vi "remove channel action.vi"(6 "user event":T1, 7 "channel":i32, 8 "error in":errorcluster, 9 "channel list":refnum<vi>, 10 "engine configuration in":refnum<class "engine configuration.lvclass">, 11 "io configuration in":refnum<class "io configuration.lvclass">) -> (0 "error out":errorcluster, 2 "engine configuration out":refnum<class "engine configuration.lvclass">, 3 "io configuration out":refnum<class "io configuration.lvclass">)   [LabVIEW 2014, in "io editor node.lvclass"]
uses:
  io editor node.lvclass
  <vilib>/NI/Configuration Framework/Controls/EventCluster.ctl
  <vilib>/NI/Configuration Framework/NISE_CEF_TreeControl.lvlib
  <vilib>/NI/Module Execution Interface/Engine Configuration/engine configuration.lvclass
  <vilib>/NI/Configuration Framework/serializable configuration/NISE_CEF_serializable configuration.lvclass
  configuration/io configuration.lvclass
  <vilib>/NI/Configuration Framework/Node/UserEventRef.ctl
  <vilib>/NI/Configuration Framework/Node/NISE_CEF_Node.lvclass
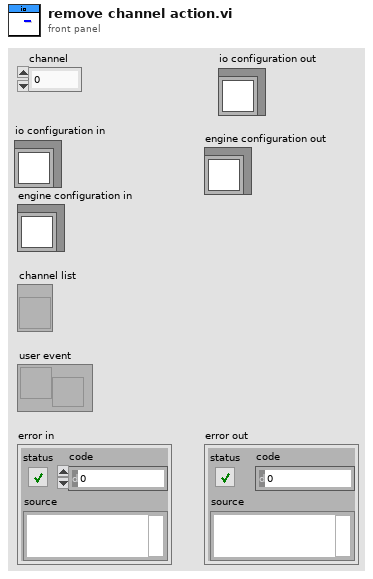
[diagram p1: front panel]
types:
  T1 = typedef "NISE_CEF_Node.lvclass/UserEventRef.ctl" = refnum<user-event>
  T2 = typedef "io editor node.lvclass/table line.ctl" = cluster{"channel":refnum<class "TBM channel.lvclass">, "tag name":string}
  T3 = typedef "NISE_CEF_TreeControl.lvlib/EventCluster.ctl" = cluster{"command":string, "data":string}
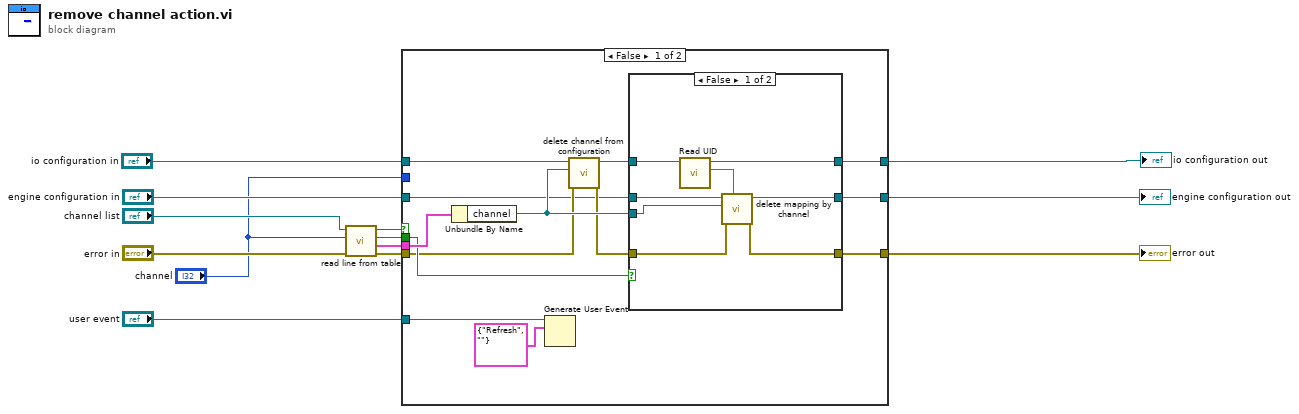
[diagram p0: block diagram]
diagram:
  n1 = call "read line from table.vi"("error in"="error in", "line number"="channel", "channels table"="channel list") -> ("error out"=w9:errorcluster, "line"=w5:T2, "empty tag?"=w8:bool, "empty channel?"=w7:bool)  [unwired: 5 in]
  n2 = case shown="False" w7 {
    tunnel: [w16 w39] -> w3
    tunnel: "channel" -> [_ _]
    tunnel: w5 -> [w26 _]
    tunnel: "io configuration in" -> [w24 w38]
    tunnel: "engine configuration in" -> [w19 w40]
    tunnel: w8 -> [w25 _]
    tunnel: w9 -> [w22 w39]
    tunnel: [w18 w40] -> w11
    tunnel: [w17 w38] -> w1
    tunnel: "user event" -> [w14 _]
    frame False {
      n3 = Unbundle By Name(w26) -> ("channel"=w23:refnum<class "TBM channel.lvclass">)
      n4 = Generate User Event(user event=w14, event data cluster=T3 {"command"="Refresh", "data"=""} ("event data")) -> ()  [unwired: 2 in, 2 out]
      n5 = call "delete channel from configuration.vi"("error in"=w22, "channel"=w23, "io configuration in"=w24) -> ("error out"=w20:errorcluster, "io configuration out"=w21:refnum<class "io configuration.lvclass">)  [unwired: 7 in]
      n6 = case shown="False" w25 {
        tunnel: w23 -> [w33 _]
        tunnel: w21 -> [w29 w35]
        tunnel: w20 -> [w32 w36]
        tunnel: w19 -> [w34 w37]
        tunnel: [w31 w37] -> w18
        tunnel: [w30 w36] -> w16
        tunnel: [w28 w35] -> w17
        frame False {
          n7 = call <vilib>:"Read UID.vi"("configuration in"=w29) -> ("instance id"=w27:string, "configuration out"=w28:refnum<class "io configuration.lvclass">)  [unwired: 8 in, 1 out]
          n8 = call <vilib>:"delete mapping by channel.vi"("owner ID"=w27, "error in"=w32, "channel"=w33, "engine configuration in"=w34) -> ("error out"=w30:errorcluster, "engine configuration out"=w31:refnum<class "engine configuration.lvclass">)  [unwired: 6 in]
        }
        frame True {
        }
      }
    }
    frame True {
    }
  }
  "engine configuration out" <- w11
  "error out" <- w3
  "io configuration out" <- w1
